vi "Control iteration 1-N.vi"(4 "Angle theta [degrees]":dbl, 6 "Number of steps":dbl, 7 "Sweep plane & fixed axis":string, 9 "Current iteration":i32, 10 "Magnetic field strength [µT]":dbl, 11 "Octant":string) -> (0 "Magnetic field z [µT]":dbl, 1 "Magnetic field y [µT]":dbl, 2 "Magnetic field x [µT]":dbl, 3 "Current angle":dbl, 5 "Output instructions 1->N":string)   [LabVIEW 2018]
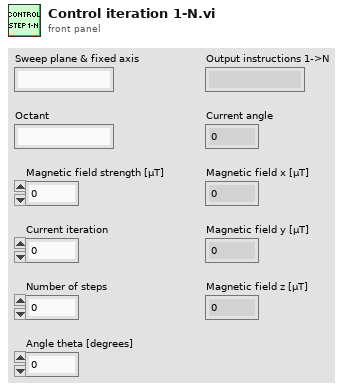
[diagram p1: front panel]
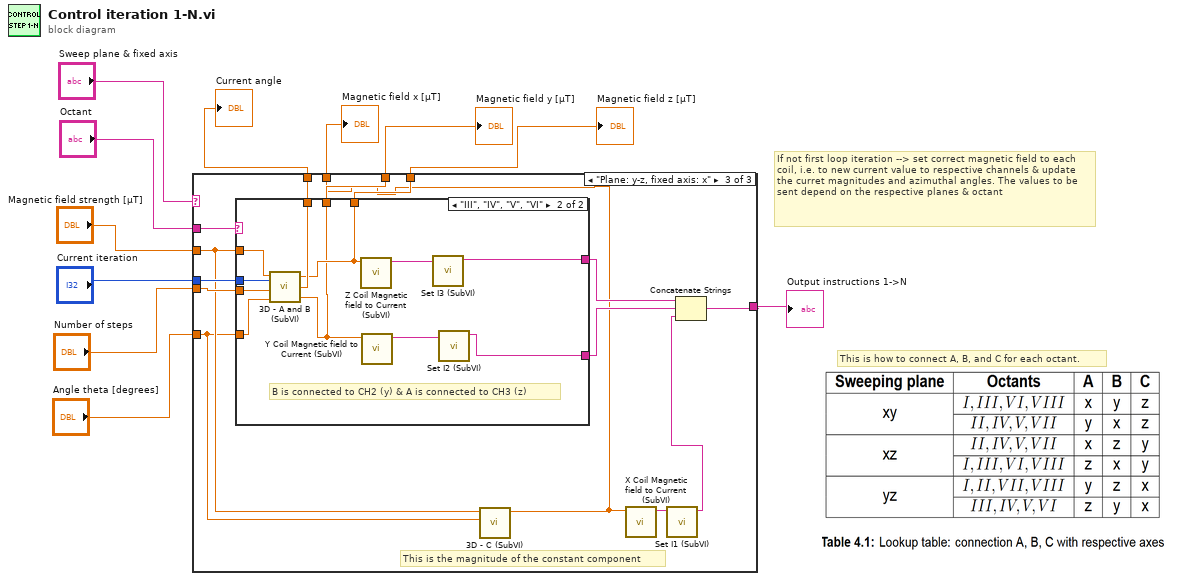
[diagram p0: block diagram]
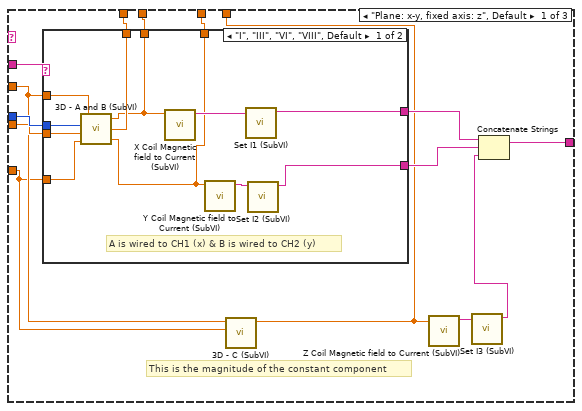
[diagram p2: hidden frame]
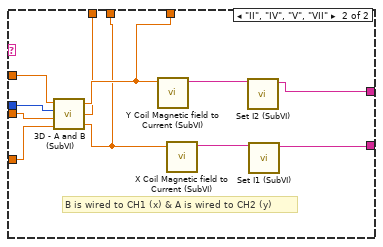
[diagram p3: hidden frame]
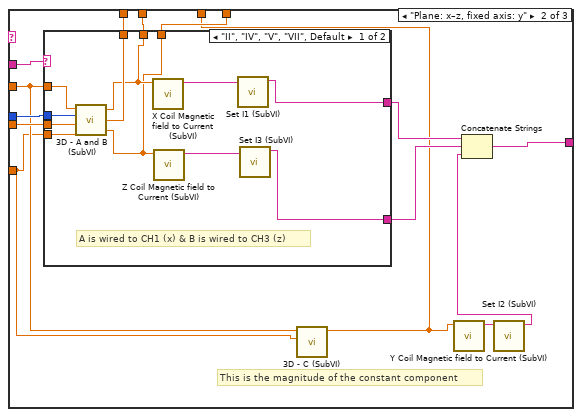
[diagram p4: hidden frame]
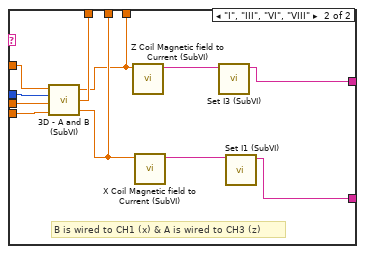
[diagram p5: hidden frame]
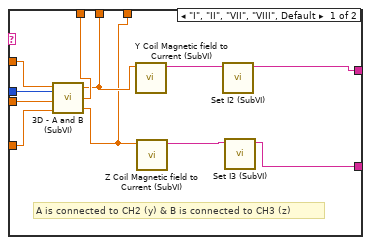
[diagram p6: hidden frame]
diagram:
  # "This is how to connect A, B, and C for each octant."
  # "If not first loop iteration --> set correct magnetic field to each coil, i.e. to new current value to respective channels & update the curret magnitudes and azimuthal angles. The values to be sent depend on the respective planes & octant"
  n1 = case shown="\"Plane: y-z, fixed axis: x\"" "Sweep plane & fixed axis" {
    tunnel: "Octant" -> [w25 w61 w97]
    tunnel: "Magnetic field strength [µT]" -> [w17 w53 w90]
    tunnel: "Current iteration" -> [w24 w57 w95]
    tunnel: "Number of steps" -> [w23 w58 w94]
    tunnel: "Angle theta [degrees]" -> [w16 w52 w89]
    tunnel: [w22 w56 w93] -> w10
    tunnel: [w19 w55 w85] -> w4
    tunnel: [w18 w49 w91] -> w3
    tunnel: [w14 w54 w92] -> w2
    tunnel: [w15 w51 w88] -> w11
    frame "Plane: x-y, fixed axis: z", Default {
      # "This is the magnitude of the constant component"
      n2 = case shown="\"I\", \"III\", \"VI\", \"VIII\", Default" w25 {
        tunnel: w17 -> [w36 w47]
        tunnel: w24 -> [w35 w46]
        tunnel: w23 -> [w34 w45]
        tunnel: w16 -> [w33 w44]
        tunnel: [w32 w37] -> w22
        tunnel: [w29 w41] -> w21
        tunnel: [w28 w39] -> w20
        tunnel: [w27 w38] -> w19
        tunnel: [w26 w43] -> w18
        frame "I", "III", "VI", "VIII", Default {
          # "A is wired to CH1 (x) & B is wired to CH2 (y)"
          n3 = call "3D - A and B (SubVI).vi"("Angle theta [degrees]"=w33, "Total steps"=w34, "Current step"=w35, "Magnitude"=w36) -> ("B_B"=w26:dbl, "Current angle"=w32:dbl, "B_A"=w27:dbl)
          n4 = call "X Coil Magnetic field to Current (SubVI).vi"("Magnetic field [µT]"=w27) -> ("Current X"=w31:string)  [unwired: 10 in]
          n5 = call "Y Coil Magnetic field to Current (SubVI).vi"("Magnetic field [µT]"=w26) -> ("Current Y"=w30:string)  [unwired: 10 in]
          n6 = call "Set I1 (SubVI).vi"("Current X"=w31) -> ("String instruction"=w29:string)  [unwired: 10 in]
          n7 = call "Set I2 (SubVI).vi"("Current Y"=w30) -> ("String"=w28:string)  [unwired: 10 in]
        }
        frame "II", "IV", "V", "VII" {
          # "B is wired to CH1 (x) & A is wired to CH2 (y)"
          n8 = call "3D - A and B (SubVI).vi"("Angle theta [degrees]"=w44, "Total steps"=w45, "Current step"=w46, "Magnitude"=w47) -> ("B_B"=w38:dbl, "Current angle"=w37:dbl, "B_A"=w43:dbl)
          n9 = call "Y Coil Magnetic field to Current (SubVI).vi"("Magnetic field [µT]"=w43) -> ("Current Y"=w42:string)  [unwired: 10 in]
          n10 = call "X Coil Magnetic field to Current (SubVI).vi"("Magnetic field [µT]"=w38) -> ("Current X"=w40:string)  [unwired: 10 in]
          n11 = call "Set I2 (SubVI).vi"("Current Y"=w42) -> ("String"=w41:string)  [unwired: 10 in]
          n12 = call "Set I1 (SubVI).vi"("Current X"=w40) -> ("String instruction"=w39:string)  [unwired: 10 in]
        }
      }
      n13 = call "3D - C (SubVI).vi"("Angle theta"=w16, "Magnitude"=w17) -> ("B_C"=w14:dbl)  [unwired: 9 in]
      n14 = call "Z Coil Magnetic field to Current (SubVI).vi"("Magnetic field [µT]"=w14) -> ("Current Z"=w13:string)  [unwired: 10 in]
      n15 = call "Set I3 (SubVI).vi"("Current Z"=w13) -> ("String"=w12:string)  [unwired: 10 in]
      n16 = Concatenate Strings(w21, w20, w12) -> (w15:string)
    }
    frame "Plane: x–z, fixed axis: y" {
      # "This is the magnitude of the constant component"
      n17 = case shown="\"II\", \"IV\", \"V\", \"VII\", Default" w61 {
        tunnel: [w64 w77] -> w60
        tunnel: [w66 w78] -> w59
        tunnel: w58 -> [w70 w83]
        tunnel: w57 -> [w71 w82]
        tunnel: w53 -> [w72 w81]
        tunnel: w52 -> [w69 w80]
        tunnel: [w68 w75] -> w56
        tunnel: [w63 w74] -> w55
        tunnel: [w62 w73] -> w54
        frame "II", "IV", "V", "VII", Default {
          # "A is wired to CH1 (x) & B is wired to CH3 (z)"
          n18 = call "3D - A and B (SubVI).vi"("Angle theta [degrees]"=w69, "Total steps"=w70, "Current step"=w71, "Magnitude"=w72) -> ("B_B"=w62:dbl, "Current angle"=w68:dbl, "B_A"=w63:dbl)
          n19 = call "X Coil Magnetic field to Current (SubVI).vi"("Magnetic field [µT]"=w63) -> ("Current X"=w67:string)  [unwired: 10 in]
          n20 = call "Z Coil Magnetic field to Current (SubVI).vi"("Magnetic field [µT]"=w62) -> ("Current Z"=w65:string)  [unwired: 10 in]
          n21 = call "Set I1 (SubVI).vi"("Current X"=w67) -> ("String instruction"=w66:string)  [unwired: 10 in]
          n22 = call "Set I3 (SubVI).vi"("Current Z"=w65) -> ("String"=w64:string)  [unwired: 10 in]
        }
        frame "I", "III", "VI", "VIII" {
          # "B is wired to CH1 (x) & A is wired to CH3 (z)"
          n23 = call "3D - A and B (SubVI).vi"("Angle theta [degrees]"=w80, "Total steps"=w83, "Current step"=w82, "Magnitude"=w81) -> ("B_B"=w74:dbl, "Current angle"=w75:dbl, "B_A"=w73:dbl)
          n24 = call "Z Coil Magnetic field to Current (SubVI).vi"("Magnetic field [µT]"=w73) -> ("Current Z"=w79:string)  [unwired: 10 in]
          n25 = call "X Coil Magnetic field to Current (SubVI).vi"("Magnetic field [µT]"=w74) -> ("Current X"=w76:string)  [unwired: 10 in]
          n26 = call "Set I3 (SubVI).vi"("Current Z"=w79) -> ("String"=w78:string)  [unwired: 10 in]
          n27 = call "Set I1 (SubVI).vi"("Current X"=w76) -> ("String instruction"=w77:string)  [unwired: 10 in]
        }
      }
      n28 = call "3D - C (SubVI).vi"("Angle theta"=w52, "Magnitude"=w53) -> ("B_C"=w49:dbl)  [unwired: 9 in]
      n29 = call "Y Coil Magnetic field to Current (SubVI).vi"("Magnetic field [µT]"=w49) -> ("Current Y"=w50:string)  [unwired: 10 in]
      n30 = call "Set I2 (SubVI).vi"("Current Y"=w50) -> ("String"=w48:string)  [unwired: 10 in]
      n31 = Concatenate Strings(w59, w60, w48) -> (w51:string)
    }
    frame "Plane: y-z, fixed axis: x" {
      # "This is the magnitude of the constant component"
      n32 = case shown="\"III\", \"IV\", \"V\", \"VI\"" w97 {
        tunnel: [w100 w109] -> w96
        tunnel: [w98 w111] -> w87
        tunnel: w90 -> [w108 w119]
        tunnel: w95 -> [w107 w118]
        tunnel: w94 -> [w106 w117]
        tunnel: w89 -> [w105 w116]
        tunnel: [w104 w115] -> w93
        tunnel: [w102 w114] -> w92
        tunnel: [w103 w113] -> w91
        frame "I", "II", "VII", "VIII", Default {
          # "A is connected to CH2 (y) & B is connected to CH3 (z)"
          n33 = call "3D - A and B (SubVI).vi"("Angle theta [degrees]"=w105, "Total steps"=w106, "Current step"=w107, "Magnitude"=w108) -> ("B_B"=w102:dbl, "Current angle"=w104:dbl, "B_A"=w103:dbl)
          n34 = call "Y Coil Magnetic field to Current (SubVI).vi"("Magnetic field [µT]"=w103) -> ("Current Y"=w101:string)  [unwired: 10 in]
          n35 = call "Z Coil Magnetic field to Current (SubVI).vi"("Magnetic field [µT]"=w102) -> ("Current Z"=w99:string)  [unwired: 10 in]
          n36 = call "Set I2 (SubVI).vi"("Current Y"=w101) -> ("String"=w100:string)  [unwired: 10 in]
          n37 = call "Set I3 (SubVI).vi"("Current Z"=w99) -> ("String"=w98:string)  [unwired: 10 in]
        }
        frame "III", "IV", "V", "VI" {
          # "B is connected to CH2 (y) & A is connected to CH3 (z)"
          n38 = call "3D - A and B (SubVI).vi"("Angle theta [degrees]"=w116, "Total steps"=w117, "Current step"=w118, "Magnitude"=w119) -> ("B_B"=w113:dbl, "Current angle"=w115:dbl, "B_A"=w114:dbl)
          n39 = call "Z Coil Magnetic field to Current (SubVI).vi"("Magnetic field [µT]"=w114) -> ("Current Z"=w110:string)  [unwired: 10 in]
          n40 = call "Y Coil Magnetic field to Current (SubVI).vi"("Magnetic field [µT]"=w113) -> ("Current Y"=w112:string)  [unwired: 10 in]
          n41 = call "Set I3 (SubVI).vi"("Current Z"=w110) -> ("String"=w109:string)  [unwired: 10 in]
          n42 = call "Set I2 (SubVI).vi"("Current Y"=w112) -> ("String"=w111:string)  [unwired: 10 in]
        }
      }
      n43 = call "3D - C (SubVI).vi"("Angle theta"=w89, "Magnitude"=w90) -> ("B_C"=w85:dbl)  [unwired: 9 in]
      n44 = call "X Coil Magnetic field to Current (SubVI).vi"("Magnetic field [µT]"=w85) -> ("Current X"=w86:string)  [unwired: 10 in]
      n45 = call "Set I1 (SubVI).vi"("Current X"=w86) -> ("String instruction"=w84:string)  [unwired: 10 in]
      n46 = Concatenate Strings(w96, w87, w84) -> (w88:string)
    }
  }
  "Output instructions 1->N" <- w11
  "Magnetic field z [µT]" <- w2
  "Magnetic field y [µT]" <- w3
  "Magnetic field x [µT]" <- w4
  "Current angle" <- w10
